vi "Ex-2 FPGA Soln.vi"() -> ()   [LabVIEW 2014]
uses:
  <userlib>/_NI SPI IP/FPGA/Controllers/Public/Transfer Settings.ctl
  <vilib>/SPI API/SPIAPI/DIO/SPI Digital IO Lines.ctl
  <vilib>/SPI API/SPIAPI/DIO/SPI DIO Enable Lines.ctl
  <vilib>/rvi/Emulation/niFpgaGetClockAttributes.vi
  <vilib>/rvi/Emulation/niFpgaSctlEmulationGetInTimedLoop.vi
  <vilib>/rvi/Emulation/niFpgaEmulationReportErrorSimple.vi
  <vilib>/rvi/Emulation/niFpgaProcessEmulError.vi
  <vilib>/rvi/interface/RandomDataEmulation/niFpgaRandomDataHandleErrors.vi
  <vilib>/rvi/Emulation/niFpgaCriticalErrorInLSC.vi
  <vilib>/rvi/DataTransferAndStorage/Container/XNode/niFpgaContainer.xnode
  <vilib>/rvi/interface/RandomDataEmulation/nirviRandomDataFpgaReadWriteTemplate.vi
  <userlib>/_NI SPI IP/FPGA/Controllers/NI SPI IP FPGA.lvlib
panel:
  in  "SPI PHY Settings":T1={"Divide Value"=10, "Transfer Length (bits)"=16, "CS Asserted Polarity"=FALSE, "Clock Polarity (CPOL)"=FALSE, "Clock Phase (CPHA)"=FALSE, "Lengthen MISO Setup"=FALSE, "Direction Change Bit"=0, "MOSI Starts as Output"=FALSE, "Tristatable MOSI"=FALSE} {"Direction Change Bit" max=64 step=1; "Transfer Length (bits)" min=1 max=64 step=1}
  out "FPGA Error":errorcluster
  out "Finished":bool
  in  "stop":bool
  out "Module Underflow":bool
  out "Acq Loop Ticks":u32
  out "DMA FIFO Full":bool
  out "Chan Count":bool
  out "First Read":bool
  in  "Number of Channels":i32=4
  in  "Acquisition Type":enum16{"Finite Samples", "Continuous Samples"}(ring)
  in  "Samps per Chan [Finite]":i32=5120
  in  "Chan Scale Array":sgl[](array[numeric])=[0.0, 0.0, 0.0, 0.0, 0.0, 0.0, 0.0, 0.0, 0.0, 0.0, 0.0, 0.0, 0.0, 0.0, 0.0, 0.0, 0.0, 0.0, 0.0, 0.0, 0.0, 0.0, 0.0, 0.0, 0.0, 0.0, 0.0, 0.0, 0.0, 0.0, 0.0, 0.0, 0.0, 0.0, 0.0, 0.0, 0.0, 0.0, 0.0, 0.0]
  out "oclk mult":u32
  out "oclk div":u32
  out "oclk freq":u32
  in  "data rate (S/s)":u32
  # "Array size fixed at 40\nelements but may be \nexpanded if needed"
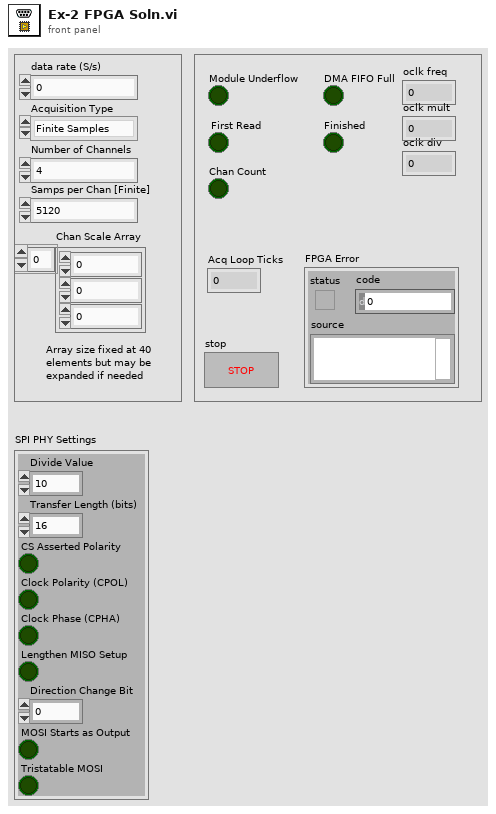
[diagram p1: front panel]
types:
  T1 = typedef "NI SPI IP FPGA.lvlib/Transfer Settings.ctl" = cluster{"Divide Value":u8, "Transfer Length (bits)":u8, "CS Asserted Polarity":bool, "Clock Polarity (CPOL)":bool, "Clock Phase (CPHA)":bool, "Lengthen MISO Setup":bool, "Direction Change Bit":u8, "MOSI Starts as Output":bool, "Tristatable MOSI":bool}
  T2 = typedef "SPI DIO Enable Lines.ctl" = cluster{"SCLK_en":refnum<k21>, "MISO_en":refnum<k21>, "MOSI_en":refnum<k21>, "CS0_en":refnum<k21>, "CS1_en":refnum<k21>, "CS2_en":refnum<k21>, "CS3_en":refnum<k21>, "CS4_en":refnum<k21>, "CS5_en":refnum<k21>}
  T3 = typedef "SPI Digital IO Lines.ctl" = cluster{"SCLK":refnum<k21>, "MISO":refnum<k21>, "MOSI":refnum<k21>, "CS 0":refnum<k21>, "CS 1":refnum<k21>, "CS 2":refnum<k21>, "CS 3":refnum<k21>, "CS 4":refnum<k21>, "CS 5":refnum<k21>}
  T4 = typedef "Internal Data (SPI API).ctl" = cluster{"DLU To SPI Engine Data FIFO":refnum<k21>, "SPI Engine to DLU Data FIFO":refnum<k21>, "Data to SPI Engine (Cache) Register":refnum<k21>, "SPI PHY Settings to SPI Engine (Cahche) Register":refnum<k21>}
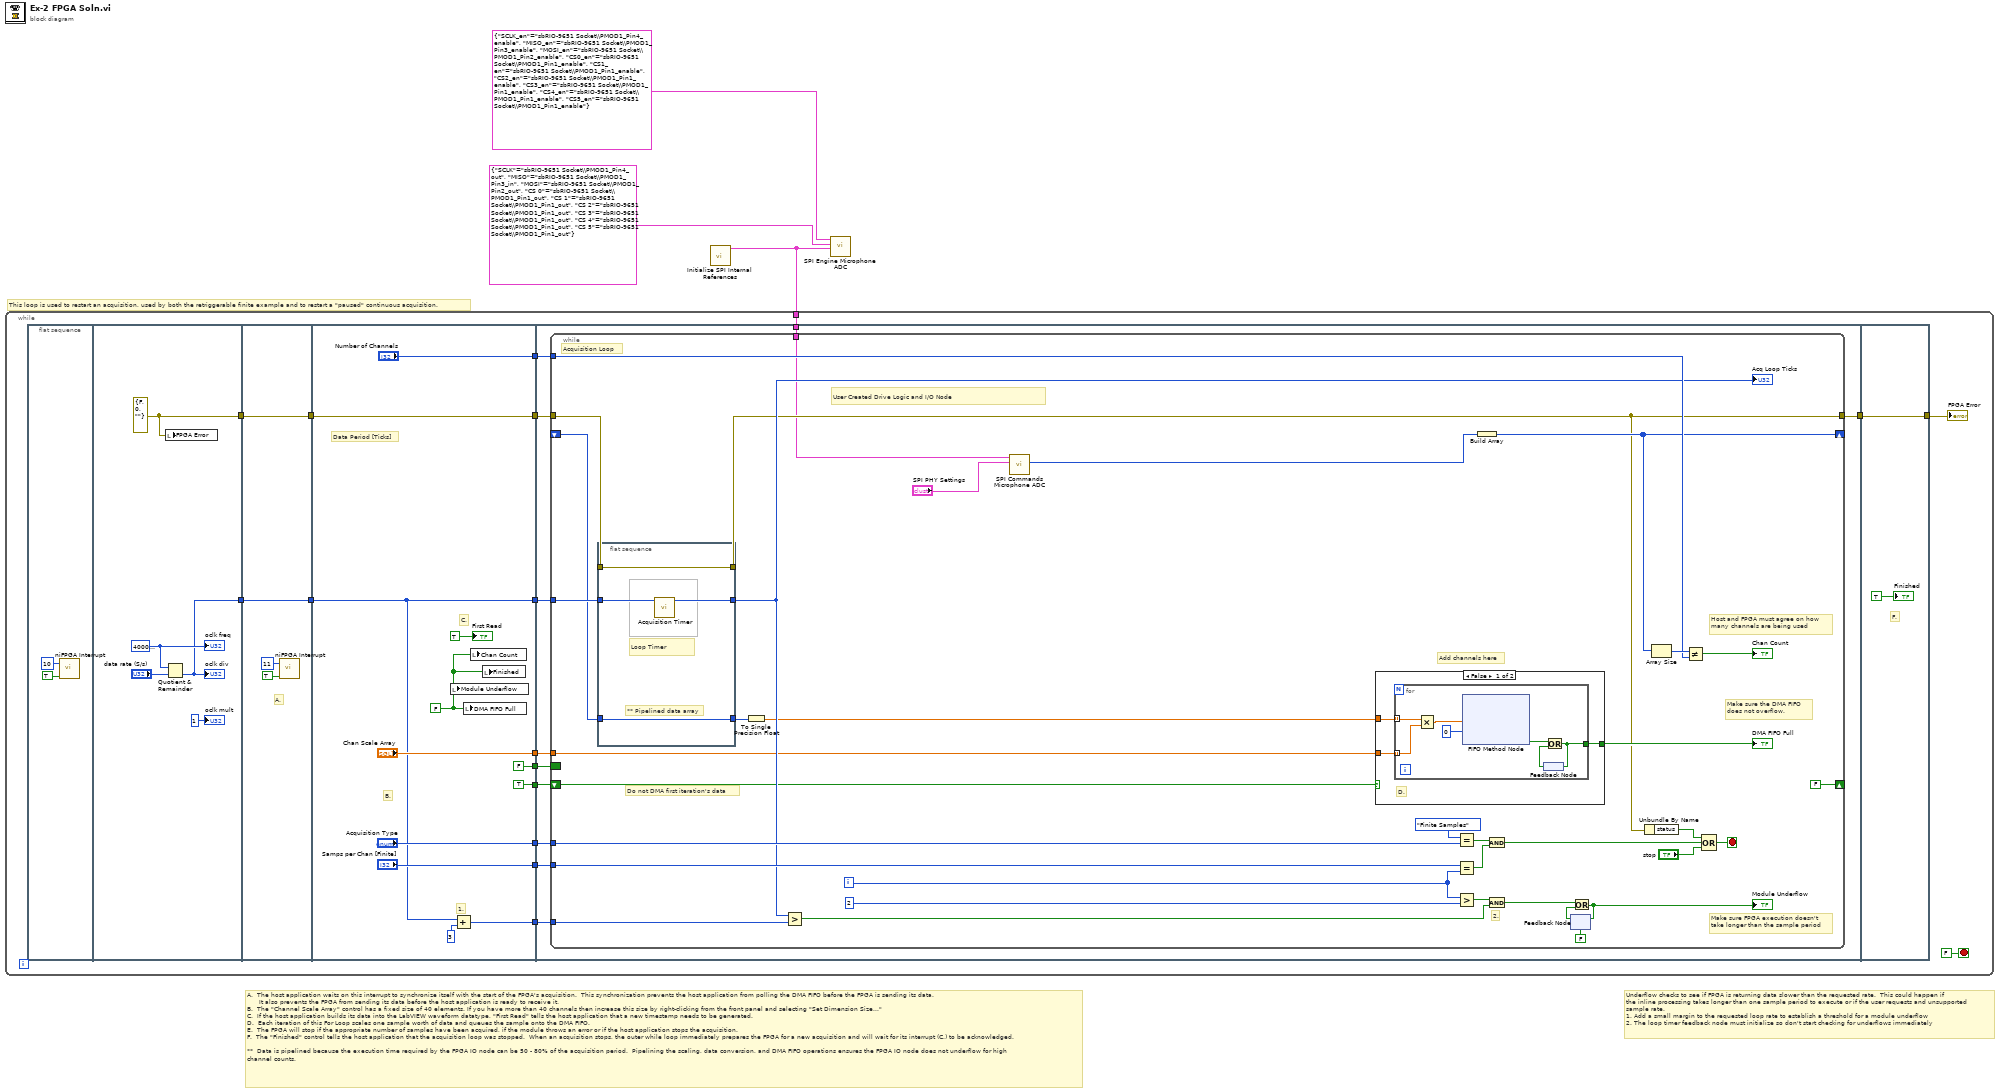
[diagram p0: block diagram]
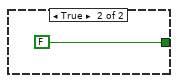
[diagram p2: hidden frame]
diagram:
  # "Underflow checks to see if FPGA is returning data slower than the requested rate.  This could happen if\nthe inline processing takes longer than one sample period to execute or if the user requests and unsupported\nsample rate.\n1. Add a small margin to the requested loop rate to establish a threshold for a module underflow \n2. The loop timer feedback node must initialize so don't start checking for underflows immediately"
  # "A.  The host application waits on this interrupt to synchronize itself with the start of the FPGA's acquisition.  This synchronization prevents the host application from polling the DMA FIFO before the FPGA is sending its data.\n      It also prevents the FPGA from sending its data before the host application is ready to receive it.\nB.  The \"Channel Scale Array\" control has a fixed size of 40 elements. If you have more than 40 channels then increase this size by right-clicking from the front panel and selecting \"Set Dimension Size...\"\nC.  If the host application builds its data into the LabVIEW waveform datatype, \"First Read\" tells the host application that a new timestamp needs to be generated.\nD.  Each iteration of this For Loop scales one sample worth of data and queues the sample onto the DMA FIFO.  \nE.  The FPGA will stop if the appropriate number of samples have been acquired, if the module throws an error or if the host application stops the acquisition.  \nF.  The \"Finished\" control tells the host application that the acquisition loop was stopped.  When an acquisition stops, the outer while loop immediately prepares the FPGA for a new acquisition and will wait for its interrupt (C.) to be acknowledged. \n\n**  Data is pipelined because the execution time required by the FPGA IO node can be 50 - 80% of the acquisition period.  Pipelining the scaling, data conversion, and DMA FIFO operations ensures the FPGA IO node does not underflow for high\nchannel counts."
  # "This loop is used to restart an acquisition, used by both the retriggerable finite example and to restart a \"paused\" continuous acquisition."
  n1 = call <vilib>:"Initialize SPI Internal References.vi"() -> ("SPI API References"=w3:T4)  [unwired: 10 in, 1 out]
  n2 = while {
    tunnel: w3 -> [w4]
    stop <- FALSE stop-if-true
    n3 = flat-sequence {
      tunnel: [w24] -> w11
      tunnel: [w23] -> w7
      tunnel: w11 -> [w29]
      tunnel: [w29] -> w10
      tunnel: [w28] -> w8
      tunnel: w7 -> [w28]
      tunnel: ["Number of Channels"] -> w20
      tunnel: ["Chan Scale Array"] -> w19
      tunnel: ["Acquisition Type"] -> w18
      tunnel: ["Samps per Chan [Finite]"] -> w17
      tunnel: [w33] -> w16
      tunnel: [w37] -> w15
      tunnel: [TRUE] -> w14
      tunnel: w10 -> [w34]
      tunnel: [w34] -> w9
      tunnel: w8 -> [w33]
      tunnel: [FALSE] -> w6
      tunnel: w20 -> [w54]
      tunnel: w19 -> [w51]
      tunnel: w18 -> [w50]
      tunnel: w17 -> [w49]
      tunnel: w16 -> [w52]
      tunnel: w15 -> [w48]
      tunnel: w14 -> [w47]
      tunnel: [w46] -> w12
      tunnel: w9 -> [w53]
      tunnel: w6 -> [w45]
      tunnel: w4 -> [w44]
      tunnel: [w106] -> w13
      tunnel: w12 -> [w106]
      frame #0 {
        n4 = call <vilib>:"niFPGA Interrupt.vi"("Wait Until Cleared (F)"=TRUE ("Wait Until Cleared"), "IRQ Number (0)"=u8 10 ("IRQ Number")) -> ()  [unwired: 1 in]
      }
      frame #1 {
        w24 = errorcluster {"status"=FALSE, "code"=0, "source"=""} ("FPGA Error")
        w25 = u32 40000000 ("oclk freq")
        n5 = Quotient & Remainder(x=w25, y="data rate (S/s)") -> (floor(x/y)=w23:u32)  [unwired: 1 out]
        "oclk div" <- w23
        n6 = local write "FPGA Error"(w24) -> ()
        "oclk mult" <- u32 1 ("oclk mult")
        "oclk freq" <- w25
      }
      frame #2 {
        # "A."
        n7 = call <vilib>:"niFPGA Interrupt.vi"("Wait Until Cleared (F)"=TRUE ("Wait Until Cleared"), "IRQ Number (0)"=u8 11 ("IRQ Number")) -> ()  [unwired: 1 in]
      }
      frame #3 {
        w42 = FALSE ("Module Underflow")
        # "Data Period [Ticks]"
        # "1."
        # "C."
        # "B."
        n8 = local write "Module Underflow"(w42) -> ()
        n9 = Add(x=w33, y=u32 3) -> (x+y=w37:u32)
        n10 = local write "DMA FIFO Full"(w42) -> ()
        n11 = local write "Chan Count"(w42) -> ()
        n12 = local write "Finished"(w42) -> ()
        "First Read" <- TRUE ("First Read")
      }
      frame #4 {
        n13 = while {
          tunnel: w50 -> [w83]
          tunnel: w49 -> [w82]
          shift-right: [w61] -> _
          shift-left: _ -> [w74]
          tunnel: w54 -> [w84]
          tunnel: w53 -> [w76]
          tunnel: [w58] -> w46
          tunnel: w52 -> [w81]
          tunnel: w48 -> [w77]
          tunnel: w51 -> [w73]
          shift-right: [FALSE] -> _
          shift-left: w47 -> [w72]
          border: w45 -> [_]
          tunnel: w44 -> [w56]
          i -> [w70]
          stop <- w88 stop-if-true
          # "User Created Drive Logic and I/O Node"
          # "Add channels here"
          # "2."
          # "Do not DMA first iteration's data"
          # "Host and FPGA must agree on how \nmany channels are being used"
          # "Acquisition Loop"
          # "Make sure the DMA FIFO\ndoes not overflow."
          # "Make sure FPGA execution doesn't\ntake longer than the sample period"
          n14 = flat-sequence {
            tunnel: w81 -> [w103]
            tunnel: [w105] -> w58
            tunnel: w76 -> [w105]
            tunnel: [w102] -> w75
            tunnel: [w104] -> w60
            tunnel: w74 -> [w104]
            frame #0 {
              # "Loop Timer"
              # "** Pipelined data array"
              n15 = call <vilib>:"Acquisition Timer.vi"("Loop Time (Ticks)"=w103) -> ("Actual Time (Ticks)"=w102:u32)  [unwired: 10 in]
            }
          }
          n16 = To Single Precision Float(number=w60) -> (single precision float=w59:sgl[])
          n17 = Greater?(x=w75, y=w77) -> (0:w80:bool)
          n18 = call "SPI Commands Microphone ADC.vi"("SPI PHY Settings"="SPI PHY Settings", "SPI API References"=w56) -> ("Data from Device"=w57:u64)  [unwired: 9 in]
          n19 = case shown="False" w72 {
            tunnel: [w93 FALSE] -> w87
            tunnel: w59 -> [w92 _]
            tunnel: w73 -> [w91 _]
            frame False {
              # "D."
              n20 = for {
                tunnel: [w99] -> w93
                tunnel: w92 -> [w98] mode=indexing
                tunnel: w91 -> [w94] mode=indexing
                n21 = Multiply(x=w98, y=w94) -> (x*y=w95:sgl)
                n22 = xnode ("FIFO Method Node")("Element"=w95, "Timeout"=0) -> ("Timed Out?"=w96:bool)  [unwired: 1 in, 1 out]
                n23 = feedback #1() -> (w100:bool)
                n24 = Or(x=w96, y=w100) -> (x .or. y?=w99:bool)
                n25 = feedback-in #1(w99) -> ()
              }
            }
            frame True {
            }
          }
          "DMA FIFO Full" <- w87
          n26 = Equal?(x=enum16{"Finite Samples", "Continuous Samples"}."Finite Samples" ("y"), y=w83) -> (x = y?=w64:bool)
          n27 = Equal?(x=w82, y=w70) -> (x = y?=w63:bool)
          n28 = Greater?(x=w70, y=2) -> (0:w79:bool)
          n29 = Build Array(w57) -> (w61:u64[])
          n30 = And(x=w64, y=w63) -> (x .and. y?=w62:bool)
          n31 = And(x=w79, y=w80) -> (x .and. y?=w66:bool)
          n32 = feedback #2(FALSE) -> (w68:bool)
          n33 = Or(x=w66, y=w68) -> (x .or. y?=w65:bool)
          "Module Underflow" <- w65
          n34 = feedback-in #2(w65) -> ()
          n35 = Unbundle By Name(w58) -> ("status"=w69:bool)
          n36 = Array Size(array=w61) -> (size(s)=w86:i32)
          n37 = Not Equal?(x=w86, y=w84) -> (x != y?=→"Chan Count":bool)
          n38 = Compound Arithmetic op=OR(w69, w62, "stop") -> (w88:bool)
          "Acq Loop Ticks" <- w75
        }
      }
      frame #5 {
        # "F."
        "Finished" <- TRUE ("Finished")
      }
    }
    "FPGA Error" <- w13
  }
  n39 = call "SPI Engine Microphone ADC.vi"("SPI API References"=w3, "SPI DIO Lines"=T3 {"SCLK"="sbRIO-9651 Socket\\PMOD1_Pin4_out", "MISO"="sbRIO-9651 Socket\\PMOD1_Pin3_in", "MOSI"="sbRIO-9651 Socket\\PMOD1_Pin2_out", "CS 0"="sbRIO-9651 Socket\\PMOD1_Pin1_out", "CS 1"="sbRIO-9651 Socket\\PMOD1_Pin1_out", "CS 2"="sbRIO-9651 Socket\\PMOD1_Pin1_out", "CS 3"="sbRIO-9651 Socket\\PMOD1_Pin1_out", "CS 4"="sbRIO-9651 Socket\\PMOD1_Pin1_out", "CS 5"="sbRIO-9651 Socket\\PMOD1_Pin1_out"}, "Enable Lines"=T2 {"SCLK_en"="sbRIO-9651 Socket\\PMOD1_Pin4_enable", "MISO_en"="sbRIO-9651 Socket\\PMOD1_Pin3_enable", "MOSI_en"="sbRIO-9651 Socket\\PMOD1_Pin2_enable", "CS0_en"="sbRIO-9651 Socket\\PMOD1_Pin1_enable", "CS1_en"="sbRIO-9651 Socket\\PMOD1_Pin1_enable", "CS2_en"="sbRIO-9651 Socket\\PMOD1_Pin1_enable", "CS3_en"="sbRIO-9651 Socket\\PMOD1_Pin1_enable", "CS4_en"="sbRIO-9651 Socket\\PMOD1_Pin1_enable", "CS5_en"="sbRIO-9651 Socket\\PMOD1_Pin1_enable"}) -> ()  [unwired: 9 in]
